vi "convert_NFProfileOL_count_to_energy.vi"(8 "exposure":dbl, 9 "divisor":dbl=52.3 format="%#_13g", 10 "offset":dbl=155.5 format="%#_13g", 11 "mean count":dbl) -> (0 "energy":dbl)   [LabVIEW 2020]
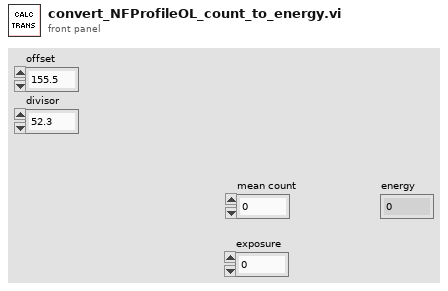
[diagram p1: front panel]
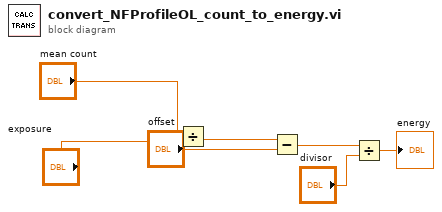
[diagram p0: block diagram]
diagram:
  n1 = Divide(x="mean count", y="exposure") -> (x/y=w5:dbl)
  n2 = Subtract(x=w5, y="offset") -> (x-y=w3:dbl)
  n3 = Divide(x=w3, y="divisor") -> (x/y=→"energy":dbl)
